vi "RC_Client 2.vi"(8 "error in (no error)":errorcluster, 11 "RC Type":T1) -> (0 "error out":errorcluster)   [LabVIEW 2019, in "RemoteControl.lvclass"]
uses:
  RemoteControl.lvclass
  <userlib>/_OpenG.lib/numeric/numeric.llb/Random Number Within Range - I32__ogtk.vi
  <userlib>/_OpenG.lib/error/error.llb/Filter Error Codes (Array)__ogtk.vi
  f0cea44e-82f5-4e56-b32e-d2cb384a2566.vi
  db51367f-c7f3-480a-b132-7f33093295d6.vi
  d8d5aeaf-e1b8-48f3-8146-827dda1e4654.vi
  Typedefs/RC Com Type--enum.ctl
panel:
  in  "milliseconds to wait":u32
  out "time (1 message) (ms)":u32
  out "startup time (ms)":u32
  out "messsages/s":dbl
  in  "remote port":u16=6341
  in  "address":string
  out "Response":string
  out "Messages":i32
  in  "Stop":bool
  out "Command reponse":string
  out "Command":string
  out "meta data\n(available commands)":string
  # "CLIENT (API)"
  # "Connection info"
  # "Message Sent"
  # "Message Received"
  # "Metrics"
  # "2"
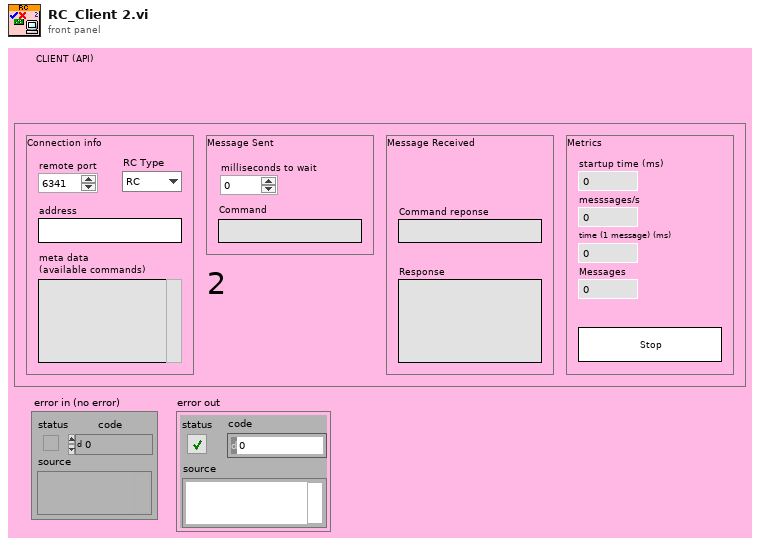
[diagram p1: front panel]
types:
  T1 = typedef "RemoteControl.lvclass/RC Com Type--enum.ctl" = enum16{"RC", "STM", "ZMQ"}
  T2 = cluster{"Command out":string, "Data out":variant, string}
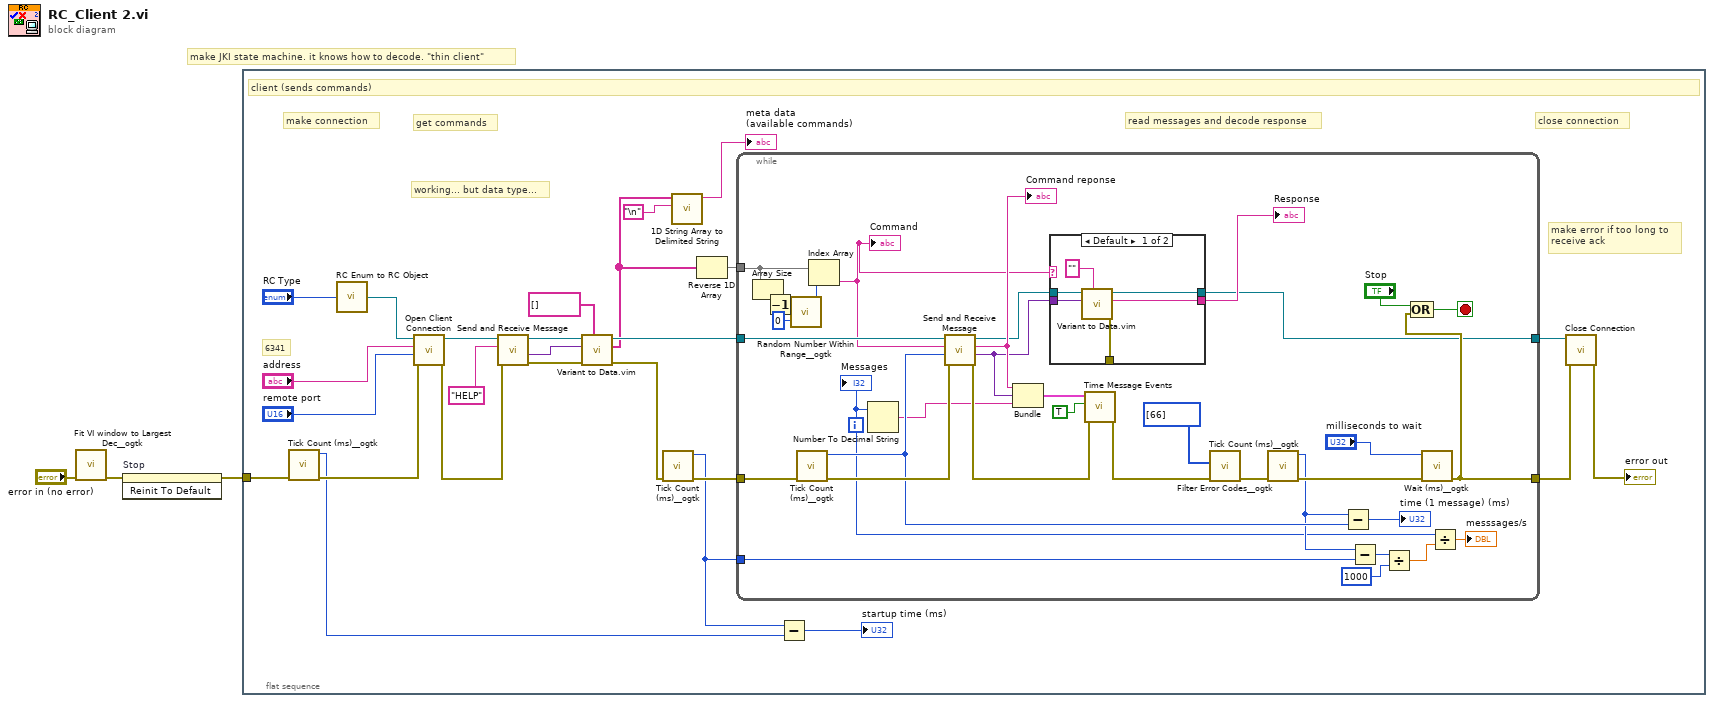
[diagram p0: block diagram]
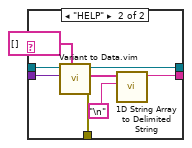
[diagram p2: hidden frame]
diagram:
  # "make JKI state machine. it knows how to decode. \"thin client\""
  n1 = call <userlib>:"Fit VI window to Largest Dec__ogtk.vi"("error in (no error)"="error in (no error)") -> ("error out"=w3:errorcluster)  [unwired: 5 in, 1 out]
  n2 = invoke on="Stop" class="Bool" method="Reinit To Default"(error in=w3) -> (error out=w2:errorcluster)  [unwired: 2 in, 2 out]
  n3 = flat-sequence {
    tunnel: w2 -> [w17]
    frame #0 {
      # "working... but data type..."
      # "close connection"
      # "read messages and decode response"
      # "get commands"
      # "make connection"
      # "6341"
      # "make error if too long to\nreceive ack"
      # "client (sends commands)"
      n4 = call <userlib>:"Tick Count (ms)__ogtk.vi"("error in (no error)"=w17) -> ("error out"=w24:errorcluster, "millisecond timer value"=w21:u32)  [unwired: 9 in]
      n5 = call "RC Enum to RC Object.vi"("RC Type"="RC Type") -> ("RemoteControl out"=w12:refnum<class "RemoteControl.lvclass">)
      n6 = call-dynamic "Open Client Connection.vi"("error in (no error)"=w24, "Port"="remote port", "address"="address", "RemoteControl in"=w12) -> ("error out"=w16:errorcluster, "RemoteControl out"=w14:refnum<class "RemoteControl.lvclass">)  [unwired: 6 in]
      n7 = call-dynamic "Send and Receive Message.vi"("error in (no error)"=w16, "Command"="HELP", "RemoteControl in"=w14) -> ("error out"=w13:errorcluster, "Data out"=w6:variant, "RemoteControl out"=w9:refnum<class "RemoteControl.lvclass">)  [unwired: 5 in, 1 out]
      n8 = call "Variant to Data.vim"("Data Type"=string[] [], "error in (no error)"=w13, "Data in"=w6, "RemoteControl in"=w9) -> ("error out"=w11:errorcluster, "Data out"=w5:string[], "RemoteControl out"=w8:refnum<class "RemoteControl.lvclass">)  [unwired: 5 in]
      n9 = call <userlib>:"Tick Count (ms)__ogtk.vi"("error in (no error)"=w11) -> ("error out"=w23:errorcluster, "millisecond timer value"=w18:u32)  [unwired: 9 in]
      n10 = call <vilib>:"1D String Array to Delimited String.vi"("delimiter"="\n", "string array"=w5) -> ("delimited string"=→"meta data\n(available commands)":string)  [unwired: 9 in]
      n11 = Reverse 1D Array(array=w5) -> (reversed array=w25:string[])
      n12 = while {
        tunnel: [w44] -> w29
        tunnel: [w33] -> w28
        tunnel: w23 -> [w58]
        tunnel: w8 -> [w62]
        tunnel: w25 -> [w48]
        tunnel: w18 -> [w38]
        i -> [w31]
        stop <- w64 stop-if-true
        n13 = Array Size(array=w48) -> (size(s)=w49:i32)
        n14 = Decrement(x=w49) -> (x-1=w47:i32)
        n15 = call-poly <userlib>:"Random Number Within Range__ogtk.vi"("High"=w47, "Low"=0) -> ("Random Number"=w51:i32)  [unwired: 3 in]
        n16 = call <userlib>:"Tick Count (ms)__ogtk.vi"("error in (no error)"=w58) -> ("error out"=w57:errorcluster, "millisecond timer value"=w45:u32)  [unwired: 9 in]
        n17 = Index Array(array=w48, index=w51) -> (element=w32:string)
        "Command" <- w32
        n18 = Number To Decimal String(number=w31) -> (decimal integer string=w30:string)  [unwired: 1 in]
        n19 = call-dynamic "Send and Receive Message.vi"("error in (no error)"=w57, "Data"=w45, "Command"=w32, "RemoteControl in"=w62) -> ("error out"=w46:errorcluster, "Data out"=w34:variant, "Command out"=w56:string, "RemoteControl out"=w35:refnum<class "RemoteControl.lvclass">)  [unwired: 4 in]
        "Command reponse" <- w56
        n20 = Bundle("Command out"=w56, "Data out"=w34, w30) -> (w55:T2)  [unwired: 1 in]
        n21 = case shown="Default" w32 {
          tunnel: [w69 w73] -> w36
          tunnel: w35 -> [w68 w77]
          tunnel: w34 -> [w67 w76]
          tunnel: [w66 w75] -> w33
          tunnel: [w65 w71] -> _
          frame Default {
            n22 = call "Variant to Data.vim"("Data Type"="", "Data in"=w67, "RemoteControl in"=w68) -> ("error out"=w65:errorcluster, "Data out"=w69:string, "RemoteControl out"=w66:refnum<class "RemoteControl.lvclass">)  [unwired: 6 in]
          }
          frame "HELP" {
            n23 = call "Variant to Data.vim"("Data Type"=string[] [], "Data in"=w76, "RemoteControl in"=w77) -> ("error out"=w71:errorcluster, "Data out"=w74:string[], "RemoteControl out"=w75:refnum<class "RemoteControl.lvclass">)  [unwired: 6 in]
            n24 = call <vilib>:"1D String Array to Delimited String.vi"("delimiter"="\n", "string array"=w74) -> ("delimited string"=w73:string)  [unwired: 9 in]
          }
        }
        "Response" <- w36
        n25 = call "Time Message Events.vi"("error in (no error)"=w46, "Debug Mode"=TRUE, "Message in"=w55) -> ("error out"=w37:errorcluster)  [unwired: 6 in, 2 out]
        n26 = call-poly <userlib>:"Filter Error Codes__ogtk.vi"("Error In"=w37, "Error Codes to Filter"=i32[] [66]) -> ("Error Out"=w61:errorcluster)  [unwired: 7 in, 2 out]
        n27 = call <userlib>:"Tick Count (ms)__ogtk.vi"("error in (no error)"=w61) -> ("error out"=w53:errorcluster, "millisecond timer value"=w40:u32)  [unwired: 9 in]
        n28 = Subtract(x=w40, y=w45) -> (x-y=→"time (1 message) (ms)":u32)
        n29 = Subtract(x=w40, y=w38) -> (x-y=w39:u32)
        n30 = Divide(x=w39, y=u32 1000) -> (x/y=w60:dbl)
        n31 = call <userlib>:"Wait (ms)__ogtk.vi"("error in (no error)"=w53, "milliseconds to wait"="milliseconds to wait") -> ("error out"=w44:errorcluster)  [unwired: 8 in, 1 out]
        n32 = Compound Arithmetic op=OR("Stop", w44) -> (w64:bool)
        n33 = Divide(x=w31, y=w60) -> (x/y=→"messsages/s":dbl)
        "Messages" <- w31
      }
      n34 = Subtract(x=w18, y=w21) -> (x-y=→"startup time (ms)":u32)
      n35 = call-dynamic "Close Connection.vi"("error in (no error)"=w29, "RemoteControl in"=w28) -> ("error out"=→"error out":errorcluster)  [unwired: 8 in, 1 out]
    }
  }
